vi "maib_save.vi"(10 "Save data":bool, 11 "Array":dbl[][](array[numeric])) -> (3 "result string":string)   [LabVIEW 2020]
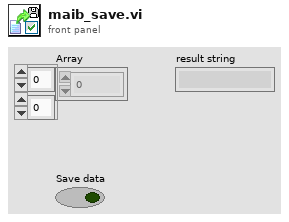
[diagram p1: front panel]
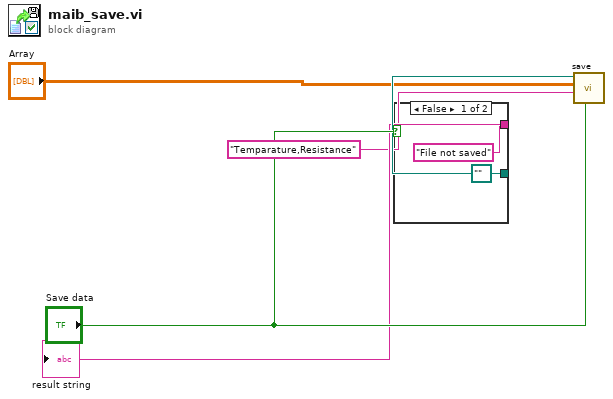
[diagram p0: block diagram]
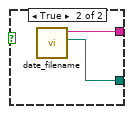
[diagram p2: hidden frame]
diagram:
  n1 = case shown="False" "Save data" {
    tunnel: ["File not saved" w9] -> w3
    tunnel: [path "" ("Path") w8] -> w4
    frame False {
    }
    frame True {
      n2 = call "date_filename.vi"() -> ("Path"=w8:path, "result string"=w9:string)  [unwired: 10 in]
    }
  }
  "result string" <- w3
  n3 = call "save.vi"("Save data"="Save data", "String"="Temparature,Resistance", "Array"="Array", "File_name"=w4) -> ()  [unwired: 8 in]
